vi "case select bl section.vi"(1 "Beamline Section":T1) -> (0 "VI Refnum":refnum<vi>)   [LabVIEW 2016, in "main.lvlib"]
uses:
  main.lvlib
  Beamline sections/beamline sections.lvlib
  Beamline sections/Low Energy End/low energy end.vi
  beamline selection.ctl
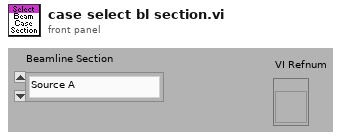
[diagram p1: front panel]
types:
  T1 = typedef "main.lvlib/beamline selection.ctl" = enum16{"Source A", "Source B", "Low Energy End", "High Energy End", "Transmission", "R30", "R45"}
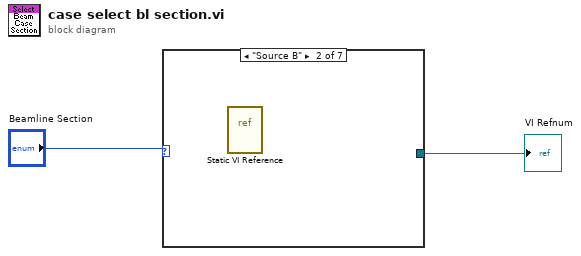
[diagram p0: block diagram]
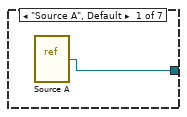
[diagram p2: hidden frame]
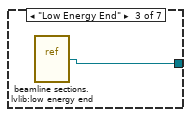
[diagram p3: hidden frame]
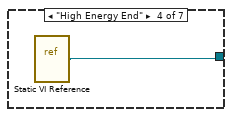
[diagram p4: hidden frame]
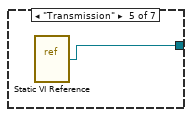
[diagram p5: hidden frame]
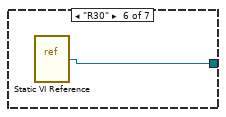
[diagram p6: hidden frame]
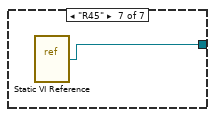
[diagram p7: hidden frame]
diagram:
  n1 = case shown="\"Source B\"" "Beamline Section" {
    tunnel: [w3 _ w4 w5 w6 w7 w8] -> w2
    frame "Source A", Default {
      n2 = vi-ref "Source A.vi"() -> (w3:refnum<vi>)
    }
    frame "Source B" {
      n3 = vi-ref "Static VI Reference"() -> ()  [unwired: 1 out]
    }
    frame "Low Energy End" {
      n4 = vi-ref "beamline sections.lvlib:low energy end.vi"() -> (w4:refnum<vi>)
    }
    frame "High Energy End" {
      n5 = vi-ref "Static VI Reference"() -> ("vi reference"=w5:refnum<vi>)
    }
    frame "Transmission" {
      n6 = vi-ref "Static VI Reference"() -> ("vi reference"=w6:refnum<vi>)
    }
    frame "R30" {
      n7 = vi-ref "Static VI Reference"() -> ("vi reference"=w7:refnum<vi>)
    }
    frame "R45" {
      n8 = vi-ref "Static VI Reference"() -> ("vi reference"=w8:refnum<vi>)
    }
  }
  "VI Refnum" <- w2
